vi "Robot Main.vi"() -> ()   [LabVIEW 2017]
doc: "Robot Main serves as the primary scheduler for your command and control robotics program. It should not be necessary to modify this VI. Instead, you should add your code to the VIs called from Robot Main - Teleop, Autonomous, and SubSystems."
uses:
  <vilib>/Rock Robotics/WPI/Camera/WPI_CameraImageSize.ctl
  <vilib>/Rock Robotics/WPI/DriverStation/WPI_DriverStationPositionInfo.ctl
  <vilib>/Rock Robotics/SystemInterfaces/NetworkCommunication/NetComm_UsageReport_ResourceType.ctl
  Framework/Robot Global Data.vi
panel:
  in  "Hook Arm Up Setpoint":dbl=1.0
  in  "Hook Arm Down Setpoint":dbl=-1.0
  in  "Climber Setpoint":dbl=-0.75
  in  "Climber Time (ms)":dbl=1000.0
  in  "Hook Up Setpoint":dbl=0.8
  in  "Hook Down Setpoint":dbl=-0.8
  in  "Autonomous Data":T1(array[cluster])=[[{"Auto Option"="Robot Left Switch Left", "Left Setpoint"=-0.8, "Right Setpoint"=-0.8, "Duration"=1600.0}, {"Auto Option"="Robot Left Switch Left", "Left Setpoint"=-1.0, "Right Setpoint"=1.0, "Duration"=450.0}, {"Auto Option"="Robot Left Switch Left", "Left Setpoint"=-0.8, "Right Setpoint"=-0.8, "Duration"=400.0}, {"Auto Option"="Robot Left Switch Left", "Left Setpoint"=0.0, "Right Setpoint"=0.0, "Duration"=0.0}, {"Auto Option"="Robot Left Switch Left", "Left Setpoint"=0.0, "Right Setpoint"=0.0, "Duration"=0.0}], [{"Auto Option"="Robot Right Switch Right", "Left Setpoint"=-0.8, "Right Setpoint"=-0.8, "Duration"=1600.0}, {"Auto Option"="Robot Right Switch Right", "Left Setpoint"=1.0, "Right Setpoint"=-1.0, "Duration"=330.0}, {"Auto Option"="Robot Right Switch Right", "Left Setpoint"=-0.8, "Right Setpoint"=-0.8, "Duration"=200.0}, {"Auto Option"="Robot Right Switch Right", "Left Setpoint"=0.0, "Right Setpoint"=0.0, "Duration"=0.0}, {"Auto Option"="Robot Right Switch Right", "Left Setpoint"=0.0, "Right Setpoint"=0.0, "Duration"=0.0}], [{"Auto Option"="Robot Left Switch Right", "Left Setpoint"=-0.8, "Right Setpoint"=-0.8, "Duration"=1600.0}, {"Auto Option"="Robot Left Switch Right", "Left Setpoint"=0.0, "Right Setpoint"=0.0, "Duration"=0.0}, {"Auto Option"="Robot Left Switch Right", "Left Setpoint"=0.0, "Right Setpoint"=0.0, "Duration"=0.0}, {"Auto Option"="Robot Left Switch Right", "Left Setpoint"=0.0, "Right Setpoint"=0.0, "Duration"=0.0}, {"Auto Option"="Robot Left Switch Right", "Left Setpoint"=0.0, "Right Setpoint"=0.0, "Duration"=0.0}], [{"Auto Option"="Robot Right Switch Left", "Left Setpoint"=-0.8, "Right Setpoint"=-0.8, "Duration"=1600.0}, {"Auto Option"="Robot Right Switch Left", "Left Setpoint"=0.0, "Right Setpoint"=0.0, "Duration"=0.0}, {"Auto Option"="Robot Right Switch Left", "Left Setpoint"=0.0, "Right Setpoint"=0.0, "Duration"=0.0}, {"Auto Option"="Robot Right Switch Left", "Left Setpoint"=0.0, "Right Setpoint"=0.0, "Duration"=0.0}, {"Auto Option"="Robot Right Switch Left", "Left Setpoint"=0.0, "Right Setpoint"=0.0, "Duration"=0.0}], [{"Auto Option"="Robot Middle Switch Left", "Left Setpoint"=-0.8, "Right Setpoint"=-0.8, "Duration"=600.0}, {"Auto Option"="Robot Middle Switch Left", "Left Setpoint"=1.0, "Right Setpoint"=-1.0, "Duration"=320.0}, {"Auto Option"="Robot Middle Switch Left", "Left Setpoint"=-0.8, "Right Setpoint"=-0.8, "Duration"=550.0}, {"Auto Option"="Robot Middle Switch Left", "Left Setpoint"=-1.0, "Right Setpoint"=1.0, "Duration"=400.0}, {"Auto Option"="Robot Middle Switch Left", "Left Setpoint"=-0.8, "Right Setpoint"=-0.8, "Duration"=650.0}], [{"Auto Option"="Robot Middle Switch Right", "Left Setpoint"=-0.8, "Right Setpoint"=-0.8, "Duration"=600.0}, {"Auto Option"="Robot Middle Switch Right", "Left Setpoint"=-1.0, "Right Setpoint"=1.0, "Duration"=400.0}, {"Auto Option"="Robot Middle Switch Right", "Left Setpoint"=-0.8, "Right Setpoint"=-0.8, "Duration"=550.0}, {"Auto Option"="Robot Middle Switch Right", "Left Setpoint"=1.0, "Right Setpoint"=-1.0, "Duration"=320.0}, {"Auto Option"="Robot Middle Switch Right", "Left Setpoint"=-0.8, "Right Setpoint"=-0.8, "Duration"=650.0}]]
  in  "Select Data Source":enum16{"auto.csv", "Robot Main"}(ring)
  in  "Auto by Time Raise Arm Time (ms)":dbl=1000.0
  in  "Auto by Time Lower Cube Time (ms)":dbl=1000.0
  in  "Auto by Time Release CubeTime (ms)":dbl=1000.0
  in  "Robot Position Selector":T2(ring)=enum."Robot Position for Debug"
  in  "Auto type":enum16{"Auto by Time", "Auto by Loops"}(ring)
  in  "Auto by Loops Raise Arm Time (ms)":dbl=1000.0
  in  "Auto by Loops Lower Cube Time (ms)":dbl=1000.0
  in  "Auto by Loops Release CubeTime (ms)":dbl=1000.0
  in  "Switch Position for debugging":string="L" caption="L = Left\nR = Right"
  in  "Robot Position for debugging":T3 caption="1 = Left\n2 = Middle\n3 = Right"
  in  "Hook Down Time (ms)":dbl=200.0
  in  "Hook Up Time (ms)":dbl=200.0
  in  "Backward Time (ms)":dbl=20.0
  in  "Forward Time (ms)":dbl=20.0
  in  "Hook Arm Down Time (ms)":dbl=200.0
  in  "Hook Arm Up Time (ms)":dbl=200.0
  in  "Right Turn Time (ms)":dbl=20.0
  in  "Left Turn Time (ms)":dbl=20.0
  in  "Rate reduction":dbl=0.9
  in  "Min Output(0 to 1)":dbl=0.8
  in  "Select Mode":T4(ring)=enum."Square with Rate"
  in  "n^x(Unbounded)":dbl=3.0 format="%#_13g"
  in  "Image Size":T5=enum."320x240"
  in  "Enable Vision":bool=TRUE
  in  "Finish":bool
  # "Joystick Sensitivity Settings"
  # "Autonomous Settings"
  # "Drive Settings"
  # "Hook Settings"
  # "Climber Settings"
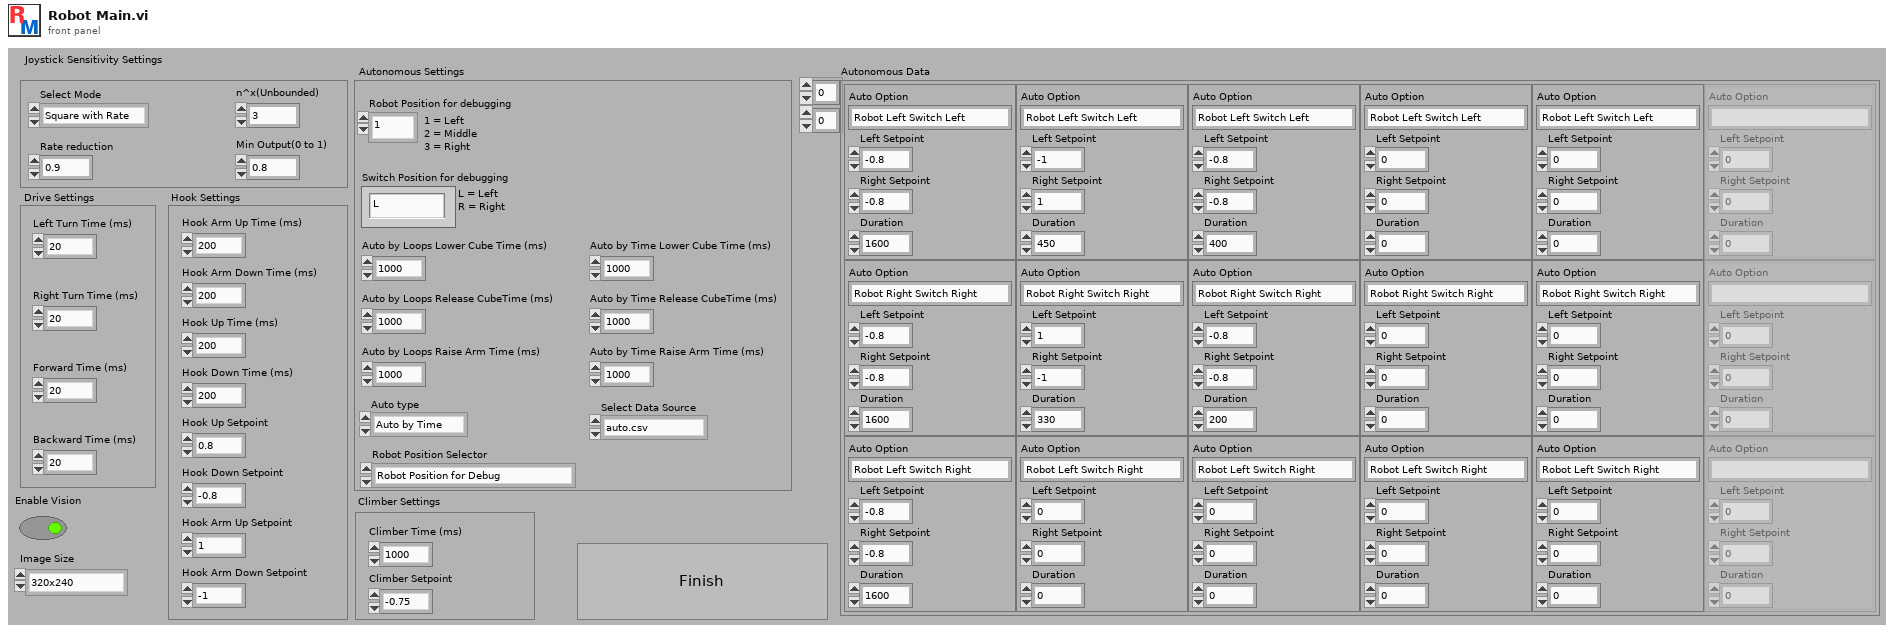
[diagram p1: front panel]
types:
  T1 = cluster{"Auto Option":string, "Left Setpoint":dbl, "Right Setpoint":dbl, "Duration":dbl}[][]
  T2 = enum16{"Robot Position from the FMS", "Robot Position from the Dashboard", "Robot Position for Debug"}
  T3 = typedef "WPI_DriverStationPositionInfo.ctl" = enum16{"1", "2", "3"}
  T4 = enum16{"Normal", "Square", "Square with Rate", "Square Root", "Linear", "Exponential"}
  T5 = typedef "WPI_CameraImageSize.ctl" = enum16{"640x480", "320x240", "160x120", "Custom"}
  T6 = typedef "NetComm_UsageReport_ResourceType.ctl" = enum8{"Controller", "Module", "Language", "CANPlugin", "Accelerometer", "ADXL345", "AnalogChannel", "AnalogTrigger", "AnalogTriggerOutput", "CANJaguar", "Compressor", "Counter", "Dashboard", "DigitalInput", "DigitalOutput", "DriverStationCIO", "DriverStationEIO", "DriverStationLCD", "Encoder", "GearTooth", "Gyro", "I2C", "Framework", "Jaguar", "Joystick", "Kinect", "KinectStick", "PIDController", "Preferences", "PWM", "Relay", "RobotDrive", "SerialPort", "Servo", "Solenoid", "SPI", "Task", "Ultrasonic", "Victor", "Button", "Command", "AxisCamera", "PCVideoServer", "SmartDashboard", "Talon", "HiTechnicColorSensor", "HiTechnicAccel", "HiTechnicCompass", "SRF08", "AnalogOutput", "Victor SP", "Talon SRX", "CAN Talon SRX", "ADXL362 Accel", "ADXRS450 Gyro", "Rev SPARK", "Mindsensors SD540", "Digital Filter", "ADIS16448", "PDP", "PCM", "PigeonIMU", "Nidec Brushless", "CTRE CANifier", "CTRE Future 0", "CTRE Future 1", "CTRE Future 2", "CTRE Future 3", "CTRE Future 4", "CTRE Future 5", "CTRE Future 6"}
  T7 = typedef "WPI_DriverStationMatch Info.ctl" = cluster{"Autonomous Elapsed Seconds":dbl, "TeleOp Elapsed Seconds":dbl, "Disabled Elapsed Seconds":dbl, "Visited Autonomous":bool, "Visited TeleOp":bool, "Visited Disabled":bool, "Autonomous Settings":cluster{"Autonomous Style":enum16{"Iterative", "Independent"}, "VI Refnum":refnum<vi>}}
  T8 = typedef "WPI_DriverStationDerivedRobotMode.ctl" = enum16{"Init", "Execute", "Stop"}
  T9 = typedef "WPI_DriverStationRobotMode2.ctl" = enum16{"Autonomous Disabled", "Autonomous Enabled", "Teleop Disabled", "Teleop Enabled", "Disconnected", "Finish", "Test Disabled", "Test Enabled", "Emergency Stopped"}
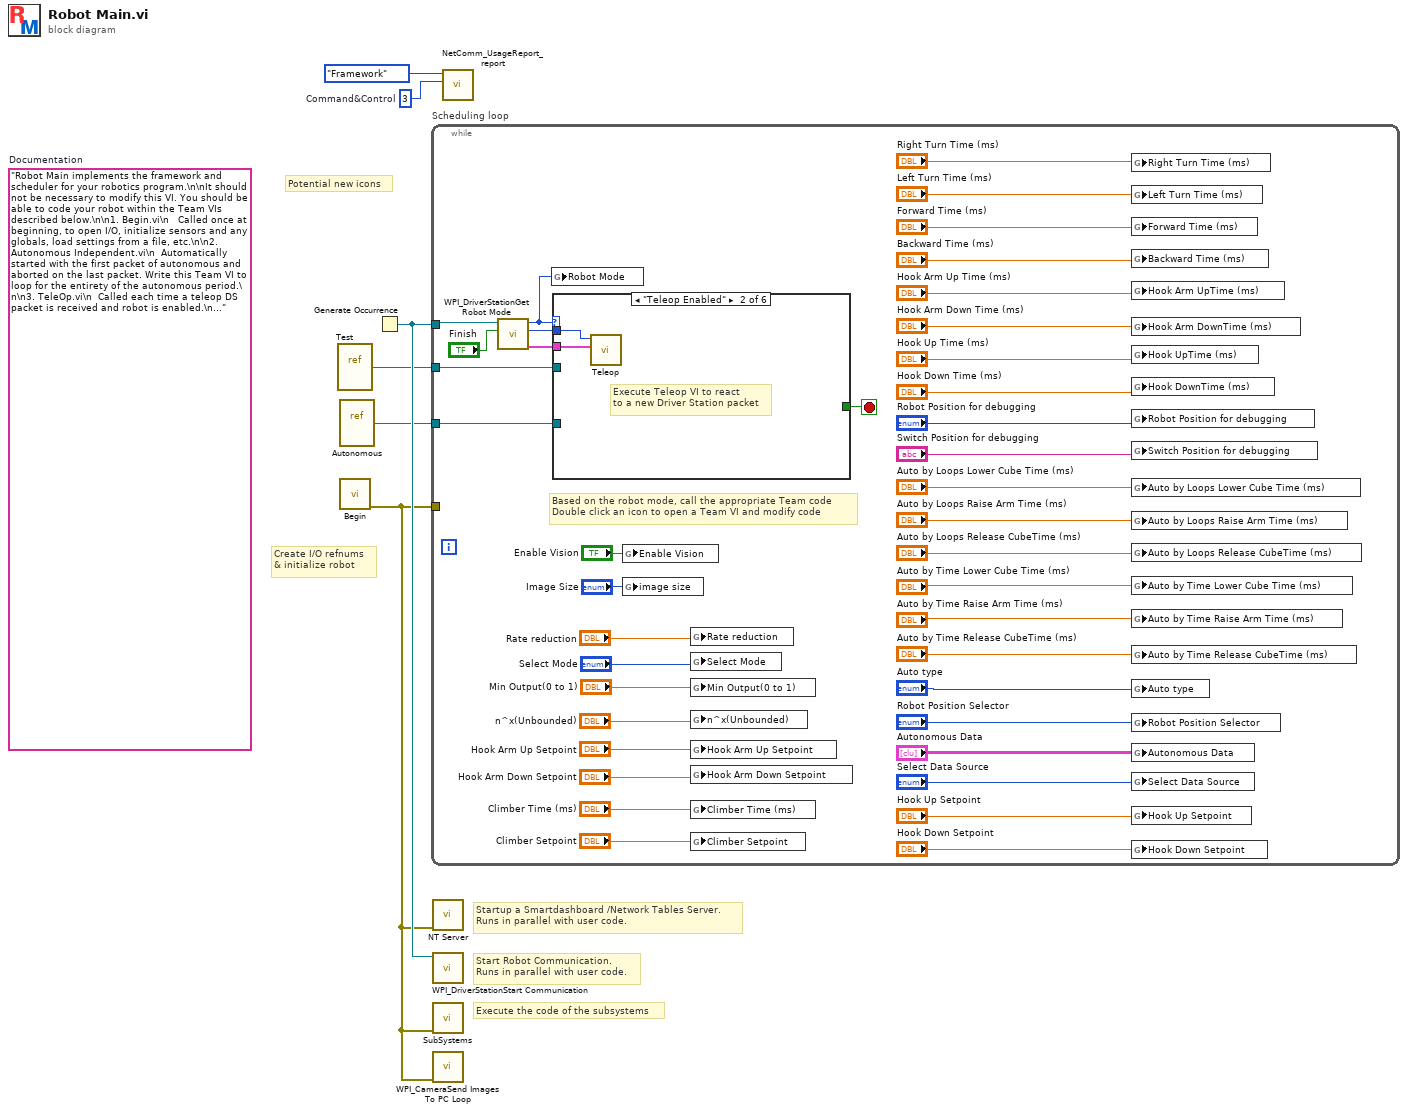
[diagram p0: block diagram]
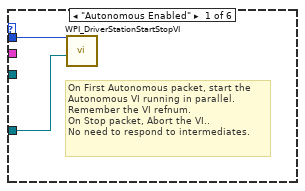
[diagram p2: hidden frame]
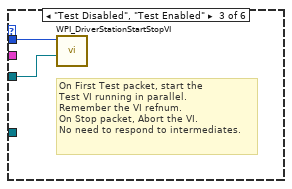
[diagram p3: hidden frame]
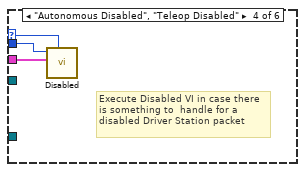
[diagram p4: hidden frame]
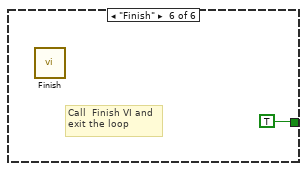
[diagram p6: hidden frame]
diagram:
  w2 = u8 3  # Command&Control
  (unwired) "Robot Main implements the framework and scheduler for your robotics program.\n\nIt should not be necessary to modify this VI. You should be able to code your robot within the Team VIs described below.\n\n1. Begin.vi\n   Called once at beginning, to open I/O, initialize sensors and any globals, load settings from a file, etc.\n\n2. Autonomous Independent.vi\n  Automatically started with the first packet of autonomous and aborted on the last packet. Write this Team VI to loop for the entirety of the autonomous period.\n\n3. TeleOp.vi\n  Called each time a teleop DS packet is received and robot is enabled.\n\n4. Disabled.vi\n  Called each time a packet is received and the robot is disabled.\n\n5. Test.vi\n  Called Automatically started with the first test packet and aborted on the last. Modify this VI to carry out robot and sensor validation tests.\n\n6. Vision.vi\n  A parallel loop that acquires and processes camera images.\n\n7. PeriodicTasks.vi\n  Parallel loops running at user-defined rates.\n\n8. Finish.vi\n  Called before exiting, so you can save data, clean up I/O, etc.\n"  # Documentation
  # "Potential new icons"
  # "Startup a Smartdashboard /Network Tables Server.\nRuns in parallel with user code."
  # "Execute the code of the subsystems"
  # "Create I/O refnums\n& initialize robot"
  # "Start Robot Communication.\nRuns in parallel with user code."
  n1 = vi-ref "Test.vi"() -> (w4:refnum<vi>)
  n2 = vi-ref "Autonomous.vi"() -> (w5:refnum<vi>)
  n3 = call "Begin.vi"() -> ("error out"=w1:errorcluster)  [unwired: 2 in, 9 out]
  n4 = Generate Occurrence() -> (w6:refnum<k4>)
  n5 = while "Scheduling loop" {
    tunnel: w6 -> [w45]
    tunnel: w1 -> [_]
    tunnel: w5 -> [w40]
    tunnel: w4 -> [w38]
    stop <- w42 stop-if-true
    # "Based on the robot mode, call the appropriate Team code\nDouble click an icon to open a Team VI and modify code"
    n6 = call <vilib>:"WPI_DriverStationGet Robot Mode.vi"("Finish"="Finish", "DS Occurrence"=w45) -> ("Match Info out"=w43:T7, "Call Context"=w46:T8, "Robot Mode"=w37:T9)  [unwired: 7 out]
    n7 = global write "Robot Global Data.vi" "Robot Mode"(w37) -> ()
    n8 = case shown="\"Teleop Enabled\"" w37 {
      selector: w37 -> [_ _ _ w53 _ _]
      tunnel: w46 -> [w48 w50 w52 w55 _ _]
      tunnel: w43 -> [_ w49 _ w54 _ _]
      tunnel: [_ _ _ _ _ TRUE] -> w42
      tunnel: w40 -> [w47 _ _ _ _ _]
      tunnel: w38 -> [_ _ w51 _ _ _]
      frame "Autonomous Enabled" {
        # "On First Autonomous packet, start the\nAutonomous VI running in parallel.\nRemember the VI refnum.\nOn Stop packet, Abort the VI..\nNo need to respond to intermediates."
        n9 = call <vilib>:"WPI_DriverStationStartStopVI.vi"("VI in"=w47, "Call Context"=w48) -> ()  [unwired: 10 in]
      }
      frame "Teleop Enabled" {
        # "Execute Teleop VI to react\nto a new Driver Station packet"
        n10 = call "Teleop.vi"("Match Info"=w49, "Call Context"=w50) -> ()  [unwired: 1 in, 9 out]
      }
      frame "Test Disabled", "Test Enabled" {
        # "On First Test packet, start the\nTest VI running in parallel.\nRemember the VI refnum.\nOn Stop packet, Abort the VI.\nNo need to respond to intermediates."
        n11 = call <vilib>:"WPI_DriverStationStartStopVI.vi"("VI in"=w51, "Call Context"=w52) -> ()  [unwired: 10 in]
      }
      frame "Autonomous Disabled", "Teleop Disabled" {
        # "Execute Disabled VI in case there\nis something to  handle for a\ndisabled Driver Station packet"
        n12 = call "Disabled.vi"("Robot Mode"=w53, "Match Info"=w54, "Call Context"=w55) -> ()  [unwired: 1 in, 8 out]
      }
      frame "Disconnected", Default {
        # "Driver Station packet didn't arrive.\nPossibly useful for diagnostics"
      }
      frame "Finish" {
        # "Call  Finish VI and\nexit the loop"
        n13 = call "Finish.vi"() -> ()  [unwired: 1 in, 7 out]
      }
    }
    n14 = global write "Robot Global Data.vi" "Enable Vision"("Enable Vision") -> ()
    n15 = global write "Robot Global Data.vi" "image size"("Image Size") -> ()
    n16 = global write "Robot Global Data.vi" "Rate reduction"("Rate reduction") -> ()
    n17 = global write "Robot Global Data.vi" "Select Mode"("Select Mode") -> ()
    n18 = global write "Robot Global Data.vi" "Min Output(0 to 1)"("Min Output(0 to 1)") -> ()
    n19 = global write "Robot Global Data.vi" "n^x(Unbounded)"("n^x(Unbounded)") -> ()
    n20 = global write "Robot Global Data.vi" "Hook Arm Up Setpoint"("Hook Arm Up Setpoint") -> ()
    n21 = global write "Robot Global Data.vi" "Hook Arm Down Setpoint"("Hook Arm Down Setpoint") -> ()
    n22 = global write "Robot Global Data.vi" "Climber Time (ms)"("Climber Time (ms)") -> ()
    n23 = global write "Robot Global Data.vi" "Climber Setpoint"("Climber Setpoint") -> ()
    n24 = global write "Robot Global Data.vi" "Right Turn Time (ms)"("Right Turn Time (ms)") -> ()
    n25 = global write "Robot Global Data.vi" "Left Turn Time (ms)"("Left Turn Time (ms)") -> ()
    n26 = global write "Robot Global Data.vi" "Forward Time (ms)"("Forward Time (ms)") -> ()
    n27 = global write "Robot Global Data.vi" "Backward Time (ms)"("Backward Time (ms)") -> ()
    n28 = global write "Robot Global Data.vi" "Hook Arm UpTime (ms)"("Hook Arm Up Time (ms)") -> ()
    n29 = global write "Robot Global Data.vi" "Hook Arm DownTime (ms)"("Hook Arm Down Time (ms)") -> ()
    n30 = global write "Robot Global Data.vi" "Hook UpTime (ms)"("Hook Up Time (ms)") -> ()
    n31 = global write "Robot Global Data.vi" "Hook DownTime (ms)"("Hook Down Time (ms)") -> ()
    n32 = global write "Robot Global Data.vi" "Robot Position for debugging"("Robot Position for debugging") -> ()
    n33 = global write "Robot Global Data.vi" "Switch Position for debugging"("Switch Position for debugging") -> ()
    n34 = global write "Robot Global Data.vi" "Auto by Loops Lower Cube Time (ms)"("Auto by Loops Lower Cube Time (ms)") -> ()
    n35 = global write "Robot Global Data.vi" "Auto by Loops Raise Arm Time (ms)"("Auto by Loops Raise Arm Time (ms)") -> ()
    n36 = global write "Robot Global Data.vi" "Auto by Loops Release CubeTime (ms)"("Auto by Loops Release CubeTime (ms)") -> ()
    n37 = global write "Robot Global Data.vi" "Auto by Time Lower Cube Time (ms)"("Auto by Time Lower Cube Time (ms)") -> ()
    n38 = global write "Robot Global Data.vi" "Auto by Time Raise Arm Time (ms)"("Auto by Time Raise Arm Time (ms)") -> ()
    n39 = global write "Robot Global Data.vi" "Auto by Time Release CubeTime (ms)"("Auto by Time Release CubeTime (ms)") -> ()
    n40 = global write "Robot Global Data.vi" "Auto type"("Auto type") -> ()
    n41 = global write "Robot Global Data.vi" "Robot Position Selector"("Robot Position Selector") -> ()
    n42 = global write "Robot Global Data.vi" "Autonomous Data"("Autonomous Data") -> ()
    n43 = global write "Robot Global Data.vi" "Select Data Source"("Select Data Source") -> ()
    n44 = global write "Robot Global Data.vi" "Hook Up Setpoint"("Hook Up Setpoint") -> ()
    n45 = global write "Robot Global Data.vi" "Hook Down Setpoint"("Hook Down Setpoint") -> ()
  }
  n46 = call <vilib>:"NT Server.vi"("error in (no error)"=w1) -> ()  [unwired: 11 in]
  n47 = call <vilib>:"WPI_DriverStationStart Communication.vi"("occurrence"=w6) -> ()  [unwired: 1 in, 10 out]
  n48 = call "SubSystems.vi"("error in"=w1) -> ()  [unwired: 11 in]
  n49 = call <vilib>:"WPI_CameraSend Images To PC Loop.vi"("error in (no error)"=w1) -> ()  [unwired: 11 in]
  n50 = call <vilib>:"NetComm_UsageReport_report.vi"("Instance Number"=w2, "Resource Type"=NetComm_UsageReport_ResourceType."Framework") -> ()  [unwired: 10 in]
